vi "Open.vi"(8 "error in (no error)":errorcluster, 9 "Explorer Visible? (F)":bool, 10 "Process Events Registration":refnum<event-registration>, 11 "Window Title":string="Action Status") -> (0 "error out":errorcluster, 2 "UI Events Registration":refnum<event-registration>)   [LabVIEW 2015, in "Simple Progress Bar.lvlib"]
uses:
  Simple Progress Bar.lvlib
  Process Events.ctl
  UI Events.ctl
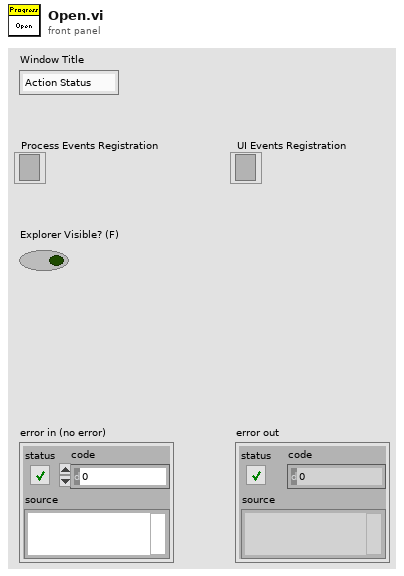
[diagram p1: front panel]
types:
  T1 = enum32{"Invalid", "Standard", "Closed", "Hidden", "Minimized", "Maximized"}
  T2 = typedef "Simple Progress Bar.lvlib/UI Events.ctl" = cluster{"Done":refnum<user-event>, "Cancel":refnum<user-event>, "Explore":refnum<user-event>}
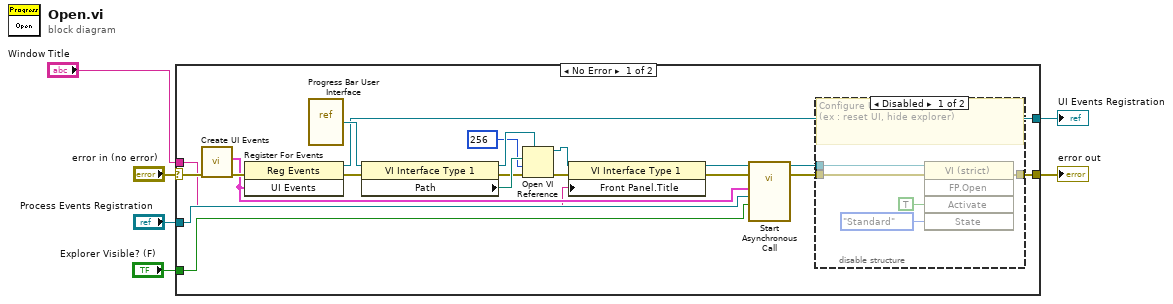
[diagram p0: block diagram]
diagram:
  n1 = case shown="No Error" "error in (no error)" {
    selector: "error in (no error)" -> [w15 w33]
    tunnel: [w20 w33] -> w5
    tunnel: [w14 _] -> w4
    tunnel: "Explorer Visible? (F)" -> [w13 _]
    tunnel: "Process Events Registration" -> [w12 _]
    tunnel: "Window Title" -> [w7 _]
    frame No Error {
      n2 = call "Create UI Events.vi"("error in (no error)"=w15) -> ("error out"=w18:errorcluster, "UI Events"=w16:T2)  [unwired: 9 in]
      n3 = register-events(error in=w18, w16) -> (reference out=w14:refnum<event-registration>, error out=w17:errorcluster)  [unwired: 1 in]
      n4 = vi-ref "Progress Bar User Interface.vi"() -> (w26:refnum<vi>)
      n5 = property class="VI Interface Type 1"(reference=w26, error in=w17) -> (reference out=w23:refnum<vi>, error out=w24:errorcluster, "Path"=w25:path)
      n6 = Open VI Reference(type specifier VI Refnum (for type only)=w23, vi path=w25, options=256, error in (no error)=w24) -> (vi reference=w9:refnum<vi>, error out=w22:errorcluster)  [unwired: 2 in]
      n7 = property class="VI Interface Type 1"(reference=w9, error in=w22, "Front Panel.Title"=w7) -> (reference out=w8:refnum<vi>, error out=w10:errorcluster)
      n8 = call-by-ref "Start Asynchronous Call"(reference=w8, error in=w10, "Explorer Visible? (F)"=w13, "Process Events Registration"=w12, "UI Events"=w16) -> (reference out=w19:refnum<vi>, error out=w21:errorcluster)  [unwired: 7 in, 2 out]
      n9 = disable-structure shown="Disabled" {
        disable-tunnel: w21 -> [w31 w32]
        disable-tunnel: [w30 w32] -> w20
        disable-tunnel: w19 -> [w29 _]
        frame Disabled {
          # "Configure UI before opening.\n(ex : reset UI, hide explorer)"
          n10 = invoke class="VI (strict)" method="FP.Open"(reference=w29, error in=w31, "Activate"=TRUE ("Activate?"), "State"=T1."Standard") -> (error out=w30:errorcluster)  [unwired: 1 in, 4 out]
        }
        frame Enabled {
        }
      }
    }
    frame Error {
    }
  }
  "error out" <- w5
  "UI Events Registration" <- w4
